vi "Write U32.vi"(7 "key":string, 8 "error in (no error)":errorcluster, 9 "default value":u32, 10 "refnum":T1, 11 "Process in":refnum<class "Process.lvclass">) -> (0 "error out":errorcluster, 1 "value":u32, 2 "refnum out":T1, 3 "Process out":refnum<class "Process.lvclass">)   [LabVIEW 2020, in "Configuration File.lvlib"]
doc: "High-level function for reading configuration file data from process class."
uses:
  Configuration File.lvlib
  Process Classes/Process/Process.lvclass
  <vilib>/Utility/config.llb/Config Data RefNum.ctl
  Process Classes/Process/Process.lvclass/Process.ctl
  <vilib>/Utility/config.llb/Write Key (U32).vi
  <vilib>/Utility/config.llb/NI_LVConfig.lvlib
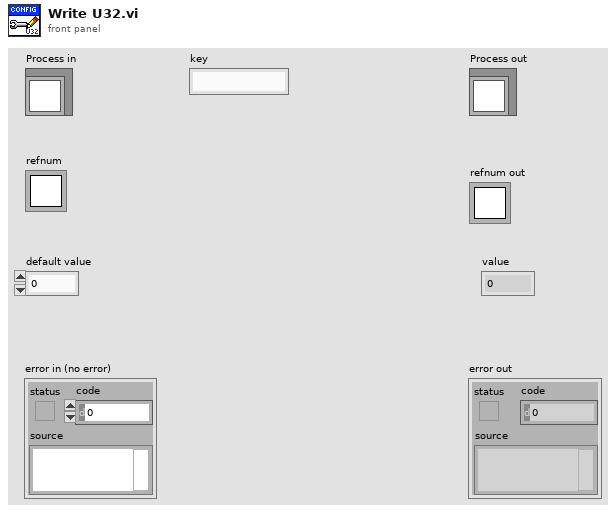
[diagram p1: front panel]
types:
  T1 = typedef "NI_LVConfig.lvlib/Config Data RefNum.ctl" = refnum<k1>
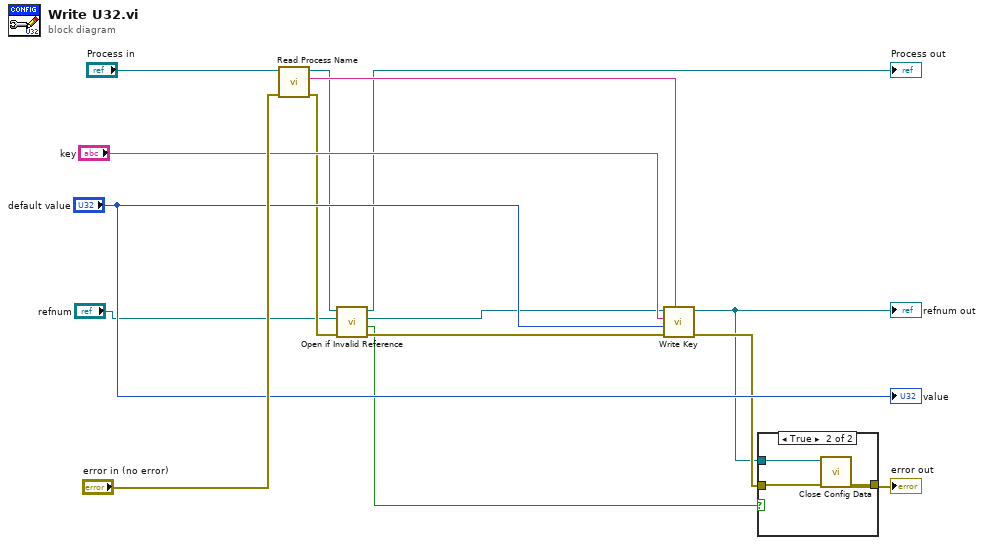
[diagram p0: block diagram]
diagram:
  n1 = call "Read Process Name.vi"("error in (no error)"="error in (no error)", "Process In"="Process in") -> ("error out"=w8:errorcluster, "Process Name"=w11:string, "Process Out"=w10:refnum<class "Process.lvclass">)  [unwired: 7 in]
  n2 = call "Open if Invalid Reference.vi"("error in (no error)"=w8, "refnum"="refnum", "Process in"=w10) -> ("error out"=w7:errorcluster, "File opened?"=w1:bool, "refnum out"=w5:T1, "Process out"=→"Process out":refnum<class "Process.lvclass">)  [unwired: 5 in]
  n3 = call-poly <vilib>:"Write Key.vi"("section"=w11, "error in (no error)"=w7, "value"="default value", "key"="key", "refnum"=w5) -> ("error out"=w3:errorcluster, "refnum out"=w2:T1)  [unwired: 4 in, 1 out]
  "refnum out" <- w2
  n4 = case shown="True" w1 {
    tunnel: w2 -> [_ w19]
    tunnel: w3 -> [w16 w18]
    tunnel: [w16 w17] -> w4
    frame False {
    }
    frame True {
      n5 = call <vilib>:"Close Config Data.vi"("error in (no error)"=w18, "refnum"=w19) -> ("error out"=w17:errorcluster)  [unwired: 8 in, 1 out]
    }
  }
  "error out" <- w4
  "value" <- "default value"
